vi "TCP.IP Client for Ripple Detection - Draft.vi"() -> ()   [LabVIEW 2021]
doc: "Demonstrates how to open a connection to an TCP server, read the data being sent, and display the data on a chart. This VI is designed to stop if the TCP connection is terminated."
panel:
  in  "File Name":path=path "F:/Career/Work/From Now/Book2.csv"
  out "Filtered":dbl[](graph)
  out "Array Size 3":u32
  out "Delayed RMS2>RMS1 for 3 data":dynamicdata(graph)
  out "RMS2>RMS1 for 3 data":dynamicdata(graph)
  out "Array Size":u32
  out "RMS2>RMS1":dynamicdata(graph)
  out "RMS1":dynamicdata(graph)
  out "RMS2":dynamicdata(graph)
  out "Raw Data Collected":dynamicdata(graph)
  in  "Boolean":bool
  in  "Server Closed":string="The server VI closed the connection."
  out "Raw Data":dbl[](graph)
  in  "Stop":bool
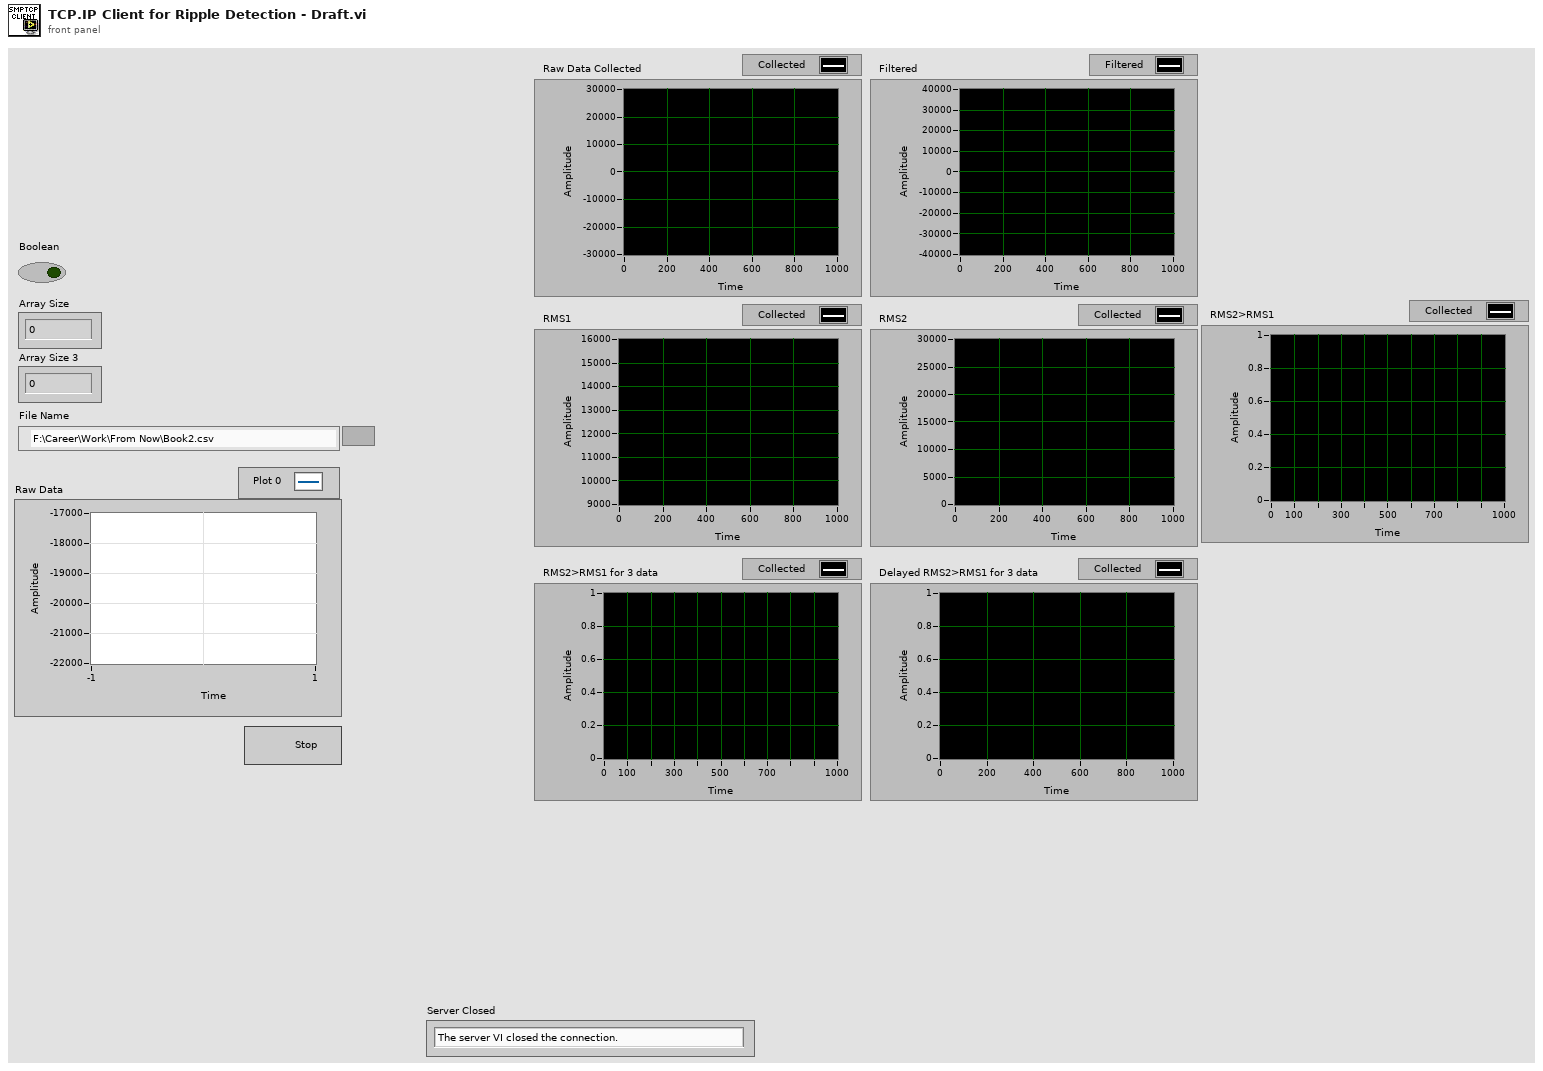
[diagram p1: front panel]
types:
  T1 = enum16{"open", "replace", "create", "open or create", "replace or create", "replace or create with confirmation"}
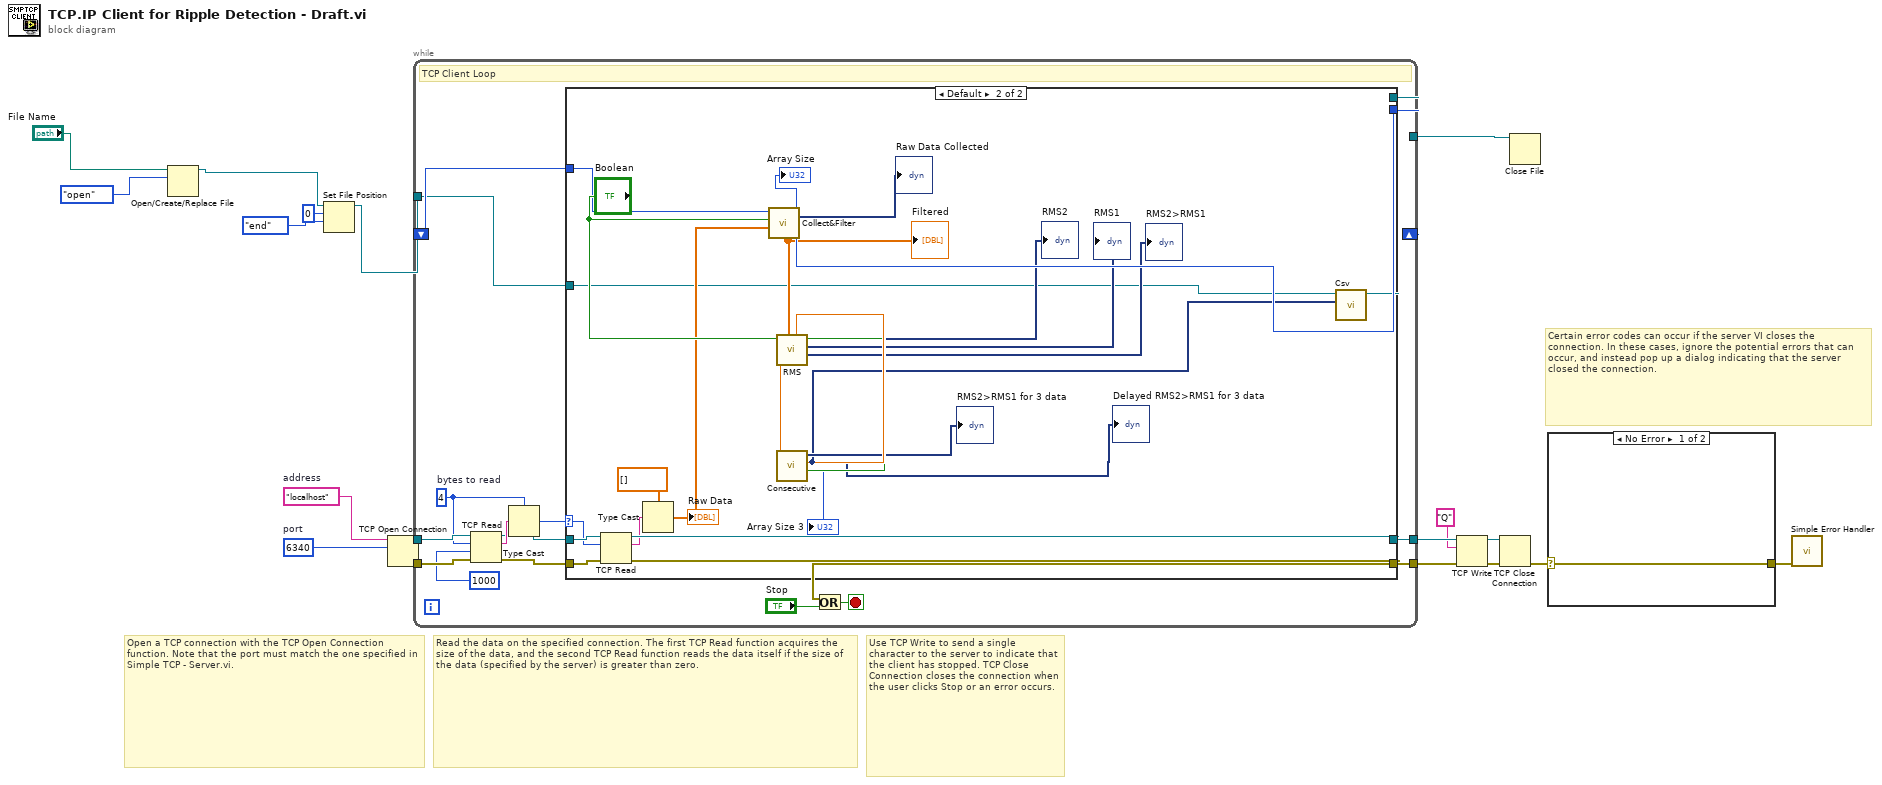
[diagram p0: block diagram]
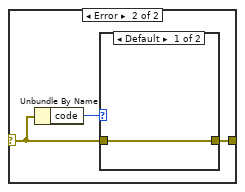
[diagram p2: hidden frame]
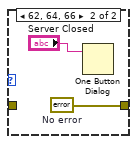
[diagram p3: hidden frame]
diagram:
  w8 = u16 6340  # port
  w9 = "localhost"  # address
  # "Certain error codes can occur if the server VI closes the connection. In these cases, ignore the potential errors that can occur, and instead pop up a dialog indicating that the server closed the connection."
  # "Use TCP Write to send a single character to the server to indicate that the client has stopped. TCP Close Connection closes the connection when the user clicks Stop or an error occurs."
  # "Read the data on the specified connection. The first TCP Read function acquires the size of the data, and the second TCP Read function reads the data itself if the size of the data (specified by the server) is greater than zero."
  # "Open a TCP connection with the TCP Open Connection function. Note that the port must match the one specified in Simple TCP - Server.vi."
  n1 = Open/Create/Replace File(file path (use dialog)="File Name", operation (0:open)=T1."open") -> (refnum out=w2:refnum<file>)  [unwired: 4 in, 2 out]
  n2 = Set File Position(offset (in bytes) (0)=i64 0, refnum=w2, from (0:start)=enum16{"start", "end", "current"}."end") -> (refnum out=w1:refnum<file>)  [unwired: 1 in, 1 out]
  n3 = TCP Open Connection(address=w9, remote port or service name=w8) -> (connection ID=w18:refnum<k5>, error out=w17:errorcluster)  [unwired: 3 in]
  n4 = while {
    tunnel: w17 -> [w30]
    tunnel: w18 -> [w31]
    tunnel: [w26] -> w15
    tunnel: [w25] -> w13
    shift-right: [w21] -> _
    shift-left: _ -> [w22]
    tunnel: [w20] -> w7
    tunnel: w1 -> [w19]
    stop <- w27 stop-if-true
    w29 = 4  # bytes to read
    # "TCP Client Loop"
    n5 = TCP Read(connection ID=w31, bytes to read=w29, error in (no error)=w30, 9:1000 ("timeout ms (25000)")) -> (connection ID out=w33:refnum<k5>, data out=w34:string, error out=w32:errorcluster)  [unwired: 1 in]
    n6 = Type Cast(type=w29, x=w34) -> (*(type *) &x=w24:i32)
    n7 = case shown="Default" w24 {
      selector: w24 -> [_ w56]
      tunnel: w33 -> [w38 w62]
      tunnel: w32 -> [w37 w61]
      tunnel: [w38 w59] -> w26
      tunnel: [w37 w58] -> w25
      tunnel: w22 -> [w36 w51]
      tunnel: [w36 w50] -> w21
      tunnel: w19 -> [w35 w40]
      tunnel: [w35 w39] -> w20
      frame ..0 {
        # "The server has not written any data"
      }
      frame Default {
        n8 = TCP Read(connection ID=w62, bytes to read=w56, error in (no error)=w61) -> (connection ID out=w59:refnum<k5>, data out=w57:string, error out=w58:errorcluster)  [unwired: 2 in]
        n9 = Type Cast(type=dbl[] [] ("chart"), x=w57) -> (*(type *) &x=w49:dbl[])
        "Raw Data" <- w49
        n10 = call "Collect&Filter.vi"("chart"=w49, "Boolean"="Boolean", "Numeric in"=w51) -> ("Collected Signals"=→"Raw Data Collected":dynamicdata, "Numeric out"=w50:i32, "Array Size"=→"Array Size":u32, "Filtered X"=w42:dbl[])  [unwired: 5 in]
        "Filtered" <- w42
        n11 = call "RMS.vi"("Filtered X"=w42) -> ("RMS2>RMS1"=→"RMS2>RMS1":dynamicdata, "RMS1"=→"RMS1":dynamicdata, "RMS2"=→"RMS2":dynamicdata, "rms value 2"=w54:dbl, "rms value"=w53:dbl)  [unwired: 6 in]
        n12 = call "Consecutive.vi"("Boolean"="Boolean", "rms value"=w53, "rms value 2"=w54) -> ("Array Size 3"=→"Array Size 3":u32, "Delayed RMS2>RMS1 for 3 data"=w41:dynamicdata, "RMS2>RMS1 for 3 data"=→"RMS2>RMS1 for 3 data":dynamicdata)  [unwired: 6 in]
        "Delayed RMS2>RMS1 for 3 data" <- w41
        n13 = call "Csv.vi"("Delayed RMS2>RMS1 for 3 data"=w41, "Byte Stream File in"=w40) -> ("Byte Stream File out"=w39:refnum<file>)  [unwired: 9 in]
      }
    }
    n14 = Or(x=w25, y="Stop") -> (x .or. y?=w27:bool)
  }
  n15 = TCP Write(connection ID=w15, data in="Q", error in (no error)=w13) -> (connection ID out=w16:refnum<k5>, error out=w14:errorcluster)  [unwired: 2 out]
  n16 = TCP Close Connection(connection ID=w16, error in (no error)=w14) -> (error out=w11:errorcluster)  [unwired: 1 in, 1 out]
  n17 = Close File(refnum=w7) -> ()  [unwired: 1 in, 2 out]
  n18 = case shown="No Error" w11 {
    selector: w11 -> [w63 w65]
    tunnel: [w63 w64] -> w10
    frame No Error {
    }
    frame Error {
      n19 = Unbundle By Name(w65) -> ("code"=w66:i32)
      n20 = case shown="Default" w66 {
        tunnel: w65 -> [w67 _]
        tunnel: [w67 w69] -> w64
        frame Default {
        }
        frame 62, 64, 66 {
          w69 = errorcluster {"status"=FALSE, "code"=0, "source"=""}  # No error
          n21 = One Button Dialog(message="Server Closed") -> ()  [unwired: 1 in, 1 out]
        }
      }
    }
  }
  n22 = call <vilib>:"Simple Error Handler.vi"("error in (no error)"=w10) -> ()  [unwired: 4 in, 5 out]
